vi "writeU8FIFO.vi"(8 "error in (no error)":errorcluster, 9 "Timeout":i32, 10 "Data":u8[](array[numeric]), 11 "IWriteU8FIFO in":refnum<class "IWriteU8FIFO.lvclass">) -> (0 "error out":errorcluster, 2 "ElementsRemaining":u32, 3 "IWriteU8FIFO out":refnum<class "IWriteU8FIFO.lvclass">)   [LabVIEW 2016, in "RTFPGA.lvlib" / "IWriteU8FIFO.lvclass"]
uses:
  IWriteU8FIFO.lvclass
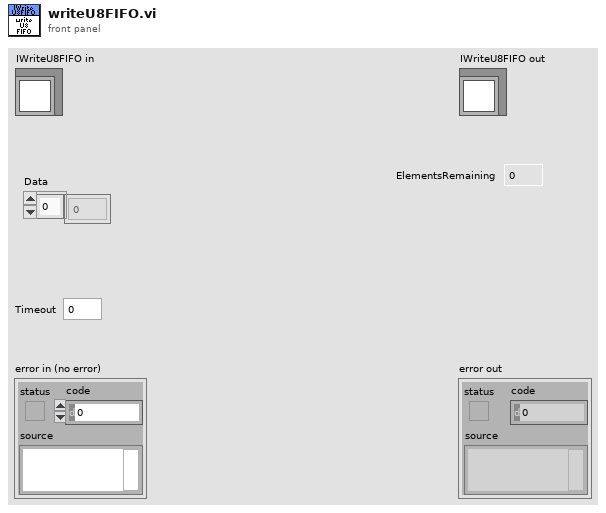
[diagram p1: front panel]
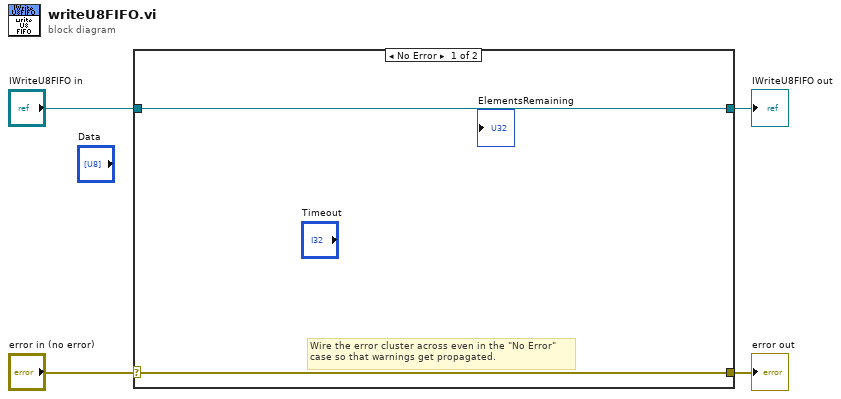
[diagram p0: block diagram]
diagram:
  n1 = case shown="No Error" "error in (no error)" {
    selector: "error in (no error)" -> [w5 w8]
    tunnel: [w5 w8] -> w3
    tunnel: [w6 w7] -> w1
    tunnel: "IWriteU8FIFO in" -> [w6 w7]
    frame No Error {
      # "Wire the error cluster across even in the \"No Error\"\ncase so that warnings get propagated."
    }
    frame Error {
    }
  }
  "error out" <- w3
  "IWriteU8FIFO out" <- w1
